vi "Read state module configuration.vi"(8 "error in":errorcluster, 11 "user tag bus module configuration In":refnum<class "user tag bus module configuration.lvclass">) -> (0 "error out":errorcluster, 2 "state module configuration":T1, 3 "user tag bus module configuration Out":refnum<class "user tag bus module configuration.lvclass">)   [LabVIEW 2013, in "user tag bus module configuration.lvclass"]
uses:
  user tag bus module configuration.lvclass
  state module configuration.ctl
  <vilib>/NI/Tag Bus Module Framework/channel/TBM channel.lvclass
  user tag bus module configuration.lvclass/user tag bus module configuration.ctl
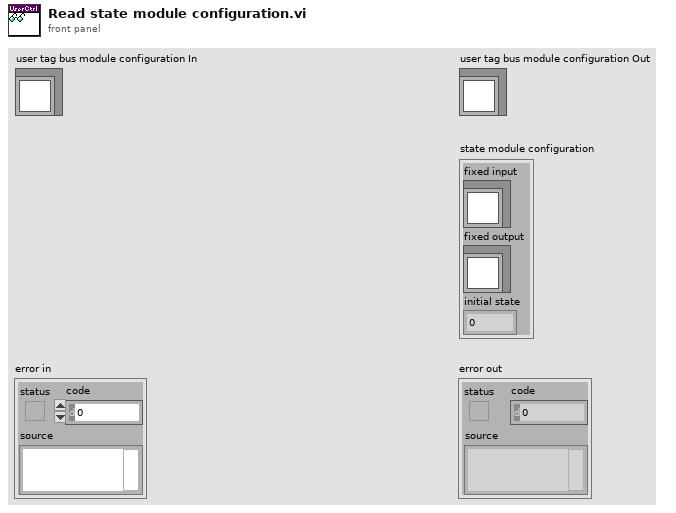
[diagram p1: front panel]
types:
  T1 = typedef "user tag bus module configuration.lvclass/state module configuration.ctl" = cluster{"fixed input":refnum<class "TBM channel.lvclass">, "fixed output":refnum<class "TBM channel.lvclass">, "initial state":u8}
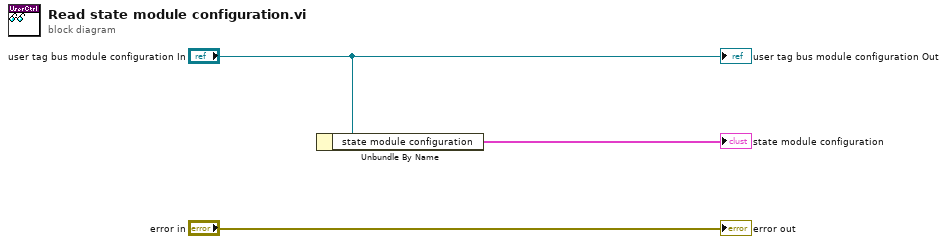
[diagram p0: block diagram]
diagram:
  n1 = Unbundle By Name("user tag bus module configuration In") -> ("state module configuration"=→"state module configuration":T1)
  "error out" <- "error in"
  "user tag bus module configuration Out" <- "user tag bus module configuration In"
